vi "Write Voffset.vi"(8 "error in (no error)":errorcluster, 10 "Voffset":dbl, 11 "Change Speaker Vparams in":refnum<class "Change Speaker Vparams.lvclass">) -> (0 "error out":errorcluster, 3 "Change Speaker Vparams out":refnum<class "Change Speaker Vparams.lvclass">)   [LabVIEW 2014, in "ePAS Library.lvlib" / "Change Speaker Vparams.lvclass"]
uses:
  Change Speaker Vparams.lvclass
  Change Speaker Vparams.lvclass/Change Speaker Vparams.ctl
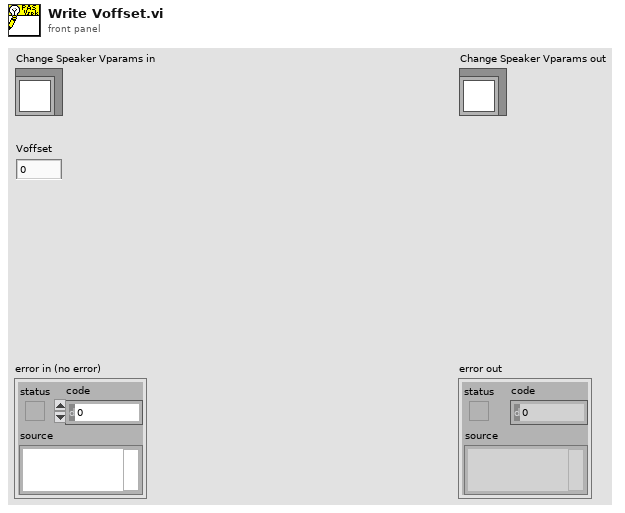
[diagram p1: front panel]
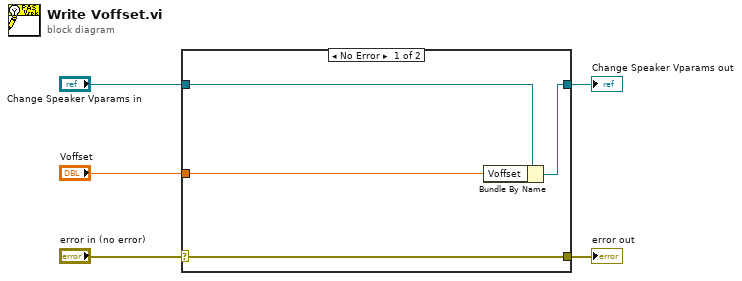
[diagram p0: block diagram]
diagram:
  n1 = case shown="No Error" "error in (no error)" {
    selector: "error in (no error)" -> [w9 w10]
    tunnel: [w9 w10] -> w4
    tunnel: [w7 w11] -> w2
    tunnel: "Change Speaker Vparams in" -> [w8 w11]
    tunnel: "Voffset" -> [w6 _]
    frame No Error {
      n2 = Bundle By Name(cluster=w8, "Voffset"=w6) -> (w7:refnum<class "Change Speaker Vparams.lvclass">)
    }
    frame Error {
    }
  }
  "error out" <- w4
  "Change Speaker Vparams out" <- w2
